vi "2D-square-lattice-generator.vi"(0 "index (row)":i32=150, 4 "Slope":dbl=41.0 format="%.2f", 5 "Period Y":dbl=333.0 format="%.2f", 6 "Spl Height":dbl=100.0 format="%.2f", 7 "Period X":dbl=329.0 format="%.2f", 8 "Width Y":dbl=200.0 format="%.2f", 9 "Width X":dbl=157.0 format="%.2f", 10 "Pixels Y":i32=1000, 11 "Pixels X":i32=1000) -> (1 "Sample Section":dbl[](graph)=[0.0, 0.0, 0.0, 0.0, 0.0, 0.0, 0.0, 0.0, 0.0, 0.0, 0.0, 0.0, 0.0, 0.0, 0.0, 0.0, 0.0, 0.0, 0.0, 0.0, 0.0, 0.0, 0.0, 0.0, 0.0, 0.0, 1.2195121951219523, 3.658536585365857, 6.0975609756097615, 8.536585365853655, 10.97560975609756, 13.414634146341465, 15.85365853658537, 18.292682926829272, 20.731707317073166, 23.17073170731707, 25.609756097560975, 28.04878048780488, 30.487804878048784, 32.92682926829268, 35.36585365853659, 37.80487804878049, 40.243902439024396, 42.6829268292683, 45.12195121951219, 47.5609756097561, 50.0, 52.4390243902439, 54.87804878048781, 57.31707317073172, 59.756097560975604, 62.19512195121951, 64.63414634146342, 67.07317073170731, 69.51219512195121, 71.95121951219512, 74.39024390243902, 76.82926829268293, 79.26829268292683, 81.70731707317074, 84.14634146341463, 86.58536585365853, 89.02439024390245, 91.46341463414635, 93.90243902439023, 96.34146341463415, 98.78048780487805, 100.0, 100.0, 100.0, 100.0, 100.0, 100.0, 100.0, 100.0, 100.0, 100.0, 100.0, 100.0, 100.0, 100.0, 100.0, 100.0, 100.0, 100.0, 100.0, 100.0, 100.0, 100.0, 100.0, 100.0, 100.0, 100.0, 100.0, 100.0, 100.0, 100.0, 100.0, 100.0, 100.0, 100.0, 100.0, 100.0, 100.0, 100.0, 100.0, 100.0, 100.0, 100.0, 100.0, 100.0, 100.0, 100.0, 100.0, 100.0, 100.0, 100.0, 100.0, 100.0, 100.0, 100.0, 100.0, 100.0, 100.0, 100.0, 100.0, 100.0, 100.0, 100.0, 100.0, 100.0, 100.0, 100.0, 100.0, 100.0, 100.0, 100.0, 100.0, 100.0, 100.0, 100.0, 100.0, 100.0, 100.0, 100.0, 100.0, 100.0, 100.0, 100.0, 100.0, 100.0, 100.0, 100.0, 100.0, 100.0, 100.0, 100.0, 100.0, 100.0, 100.0, 100.0, 100.0, 100.0, 100.0, 100.0, 100.0, 100.0, 100.0, 100.0, 100.0, 100.0, 100.0, 100.0, 100.0, 100.0, 100.0, 100.0, 100.0, 100.0, 100.0, 100.0, 100.0, 100.0, 100.0, 100.0, 100.0, 100.0, 100.0, 100.0, 100.0, 100.0, 100.0, 100.0, 100.0, 100.0, 100.0, 100.0, 100.0, 100.0, 100.0, 100.0, 100.0, 100.0, 100.0, 100.0, 100.0, 100.0, 100.0, 100.0, 100.0, 100.0, 100.0, 100.0, 100.0, 100.0, 100.0, 100.0, 100.0, 100.0, 100.0, 100.0, 100.0, 100.0, 100.0, 100.0, 100.0, 100.0, 100.0, 100.0, 100.0, 100.0, 100.0, 100.0, 100.0, 100.0, 100.0, 100.0, 100.0, 100.0, 100.0, 100.0, 100.0, 100.0, 100.0, 100.0, 100.0, 100.0, 100.0, 100.0, 100.0, 100.0, 100.0, 100.0, 100.0, 100.0, 100.0, 100.0, 100.0, 100.0, 100.0, 100.0, 100.0, 100.0, 100.0, 100.0, 100.0, 100.0, 98.78048780487805, 96.34146341463415, 93.90243902439023, 91.46341463414635, 89.02439024390245, 86.58536585365853, 84.14634146341463, 81.70731707317074, 79.26829268292683, 76.82926829268293, 74.39024390243902, 71.95121951219512, 69.51219512195121, 67.07317073170731, 64.63414634146342, 62.19512195121951, 59.756097560975604, 57.31707317073172, 54.87804878048781, 52.4390243902439, 50.0, 47.5609756097561, 45.12195121951219, 42.6829268292683, 40.243902439024396, 37.80487804878049, 35.36585365853659, 32.92682926829268, 30.487804878048784, 28.04878048780488, 25.609756097560975, 23.17073170731707, 20.731707317073166, 18.292682926829272, 15.85365853658537, 13.414634146341465, 10.97560975609756, 8.536585365853655, 6.0975609756097615, 3.658536585365857, 1.2195121951219523, 0.0, 0.0, 0.0, 0.0, 0.0, 0.0, 0.0, 0.0, 0.0, 0.0, 0.0, 0.0, 0.0, 0.0, 0.0, 0.0, 0.0, 0.0, 0.0, 0.0, 0.0, 0.0, 0.0, 0.0, 0.0, 0.0, 0.0, 0.0, 0.0, 0.0, 0.0, 0.0, 0.0, 0.0, 0.0, 0.0, 0.0, 0.0, 0.0, 0.0, 0.0, 0.0, 0.0, 0.0, 0.0, 0.0, 0.0, 0.0, 0.0, 0.0, 0.0, 1.2195121951219523, 3.658536585365857, 6.0975609756097615, 8.536585365853655, 10.97560975609756, 13.414634146341465, 15.85365853658537, 18.292682926829272, 20.731707317073166, 23.17073170731707, 25.609756097560975, 28.04878048780488, 30.487804878048784, 32.92682926829268, 35.36585365853659, 37.80487804878049, 40.243902439024396, 42.6829268292683, 45.12195121951219, 47.5609756097561, 50.0, 52.4390243902439, 54.87804878048781, 57.31707317073172, 59.756097560975604, 62.19512195121951, 64.63414634146342, 67.07317073170731, 69.51219512195121, 71.95121951219512, 74.39024390243902, 76.82926829268293, 79.26829268292683, 81.70731707317074, 84.14634146341463, 86.58536585365853, 89.02439024390245, 91.46341463414635, 93.90243902439023, 96.34146341463415, 98.78048780487805, 100.0, 100.0, 100.0, 100.0, 100.0, 100.0, 100.0, 100.0, 100.0, 100.0, 100.0, 100.0, 100.0, 100.0, 100.0, 100.0, 100.0, 100.0, 100.0, 100.0, 100.0, 100.0, 100.0, 100.0, 100.0, 100.0, 100.0, 100.0, 100.0, 100.0, 100.0, 100.0, 100.0, 100.0, 100.0, 100.0, 100.0, 100.0, 100.0, 100.0, 100.0, 100.0, 100.0, 100.0, 100.0, 100.0, 100.0, 100.0, 100.0, 100.0, 100.0, 100.0, 100.0, 100.0, 100.0, 100.0, 100.0, 100.0, 100.0, 100.0, 100.0, 100.0, 100.0, 100.0, 100.0, 100.0, 100.0, 100.0, 100.0, 100.0, 100.0, 100.0, 100.0, 100.0, 100.0, 100.0, 100.0, 100.0, 100.0, 100.0, 100.0, 100.0, 100.0, 100.0, 100.0, 100.0, 100.0, 100.0, 100.0, 100.0, 100.0, 100.0, 100.0, 100.0, 100.0, 100.0, 100.0, 100.0, 100.0, 100.0, 100.0, 100.0, 100.0, 100.0, 100.0, 100.0, 100.0, 100.0, 100.0, 100.0, 100.0, 100.0, 100.0, 100.0, 100.0, 100.0, 100.0, 100.0, 100.0, 100.0, 100.0, 100.0, 100.0, 100.0, 100.0, 100.0, 100.0, 100.0, 100.0, 100.0, 100.0, 100.0, 100.0, 100.0, 100.0, 100.0, 100.0, 100.0, 100.0, 100.0, 100.0, 100.0, 100.0, 100.0, 100.0, 100.0, 100.0, 100.0, 100.0, 100.0, 100.0, 100.0, 100.0, 100.0, 100.0, 100.0, 100.0, 100.0, 100.0, 100.0, 100.0, 100.0, 100.0, 100.0, 100.0, 100.0, 100.0, 100.0, 100.0, 100.0, 100.0, 100.0, 100.0, 100.0, 100.0, 100.0, 100.0, 100.0, 100.0, 100.0, 100.0, 100.0, 100.0, 100.0, 100.0, 100.0, 100.0, 100.0, 100.0, 100.0, 100.0, 100.0, 100.0, 100.0, 100.0, 100.0, 100.0, 100.0, 100.0, 100.0, 98.78048780487805, 96.34146341463415, 93.90243902439023, 91.46341463414635, 89.02439024390245, 86.58536585365853, 84.14634146341463, 81.70731707317074, 79.26829268292683, 76.82926829268293, 74.39024390243902, 71.95121951219512, 69.51219512195121, 67.07317073170731, 64.63414634146342, 62.19512195121951, 59.756097560975604, 57.31707317073172, 54.87804878048781, 52.4390243902439, 50.0, 47.5609756097561, 45.12195121951219, 42.6829268292683, 40.243902439024396, 37.80487804878049, 35.36585365853659, 32.92682926829268, 30.487804878048784, 28.04878048780488, 25.609756097560975, 23.17073170731707, 20.731707317073166, 18.292682926829272, 15.85365853658537, 13.414634146341465, 10.97560975609756, 8.536585365853655, 6.0975609756097615, 3.658536585365857, 1.2195121951219523, 0.0, 0.0, 0.0, 0.0, 0.0, 0.0, 0.0, 0.0, 0.0, 0.0, 0.0, 0.0, 0.0, 0.0, 0.0, 0.0, 0.0, 0.0, 0.0, 0.0, 0.0, 0.0, 0.0, 0.0, 0.0, 0.0, 0.0, 0.0, 0.0, 0.0, 0.0, 0.0, 0.0, 0.0, 0.0, 0.0, 0.0, 0.0, 0.0, 0.0, 0.0, 0.0, 0.0, 0.0, 0.0, 0.0, 0.0, 0.0, 0.0, 0.0, 0.0, 1.2195121951219523, 3.658536585365857, 6.0975609756097615, 8.536585365853655, 10.97560975609756, 13.414634146341465, 15.85365853658537, 18.292682926829272, 20.731707317073166, 23.17073170731707, 25.609756097560975, 28.04878048780488, 30.487804878048784, 32.92682926829268, 35.36585365853659, 37.80487804878049, 40.243902439024396, 42.6829268292683, 45.12195121951219, 47.5609756097561, 50.0, 52.4390243902439, 54.87804878048781, 57.31707317073172, 59.756097560975604, 62.19512195121951, 64.63414634146342, 67.07317073170731, 69.51219512195121, 71.95121951219512, 74.39024390243902, 76.82926829268293, 79.26829268292683, 81.70731707317074, 84.14634146341463, 86.58536585365853, 89.02439024390245, 91.46341463414635, 93.90243902439023, 96.34146341463415, 98.78048780487805, 100.0, 100.0, 100.0, 100.0, 100.0, 100.0, 100.0, 100.0, 100.0, 100.0, 100.0, 100.0, 100.0, 100.0, 100.0, 100.0, 100.0, 100.0, 100.0, 100.0, 100.0, 100.0, 100.0, 100.0, 100.0, 100.0, 100.0, 100.0, 100.0, 100.0, 100.0, 100.0, 100.0, 100.0, 100.0, 100.0, 100.0, 100.0, 100.0, 100.0, 100.0, 100.0, 100.0, 100.0, 100.0, 100.0, 100.0, 100.0, 100.0, 100.0, 100.0, 100.0, 100.0, 100.0, 100.0, 100.0, 100.0, 100.0, 100.0, 100.0, 100.0, 100.0, 100.0, 100.0, 100.0, 100.0, 100.0, 100.0, 100.0, 100.0, 100.0, 100.0, 100.0, 100.0, 100.0, 100.0, 100.0, 100.0, 100.0, 100.0, 100.0, 100.0, 100.0, 100.0, 100.0, 100.0, 100.0, 100.0, 100.0, 100.0, 100.0, 100.0, 100.0, 100.0, 100.0, 100.0, 100.0, 100.0, 100.0, 100.0, 100.0, 100.0, 100.0, 100.0, 100.0, 100.0, 100.0, 100.0, 100.0, 100.0, 100.0, 100.0, 100.0, 100.0, 100.0, 100.0, 100.0, 100.0, 100.0, 100.0, 100.0, 100.0, 100.0, 100.0, 100.0, 100.0, 100.0, 100.0, 100.0, 100.0, 100.0, 100.0, 100.0, 100.0, 100.0, 100.0, 100.0, 100.0, 100.0, 100.0, 100.0, 100.0, 100.0, 100.0, 100.0, 100.0, 100.0, 100.0, 100.0, 100.0, 100.0, 100.0, 100.0, 100.0, 100.0, 100.0, 100.0, 100.0, 100.0, 100.0, 100.0, 100.0, 100.0, 100.0, 100.0, 100.0, 100.0, 100.0, 100.0, 100.0, 100.0, 100.0, 100.0, 100.0, 100.0, 100.0, 100.0, 100.0, 100.0, 100.0, 100.0, 100.0, 100.0, 100.0, 100.0, 100.0, 100.0, 100.0, 100.0, 100.0, 100.0, 100.0, 100.0, 100.0, 100.0, 100.0, 100.0, 100.0, 100.0, 100.0, 98.78048780487805, 96.34146341463415, 93.90243902439023, 91.46341463414635, 89.02439024390245, 86.58536585365853, 84.14634146341463, 81.70731707317074, 79.26829268292683, 76.82926829268293, 74.39024390243902, 71.95121951219512, 69.51219512195121, 67.07317073170731, 64.63414634146342, 62.19512195121951, 59.756097560975604, 57.31707317073172, 54.87804878048781, 52.4390243902439, 50.0, 47.5609756097561, 45.12195121951219, 42.6829268292683, 40.243902439024396, 37.80487804878049, 35.36585365853659, 32.92682926829268, 30.487804878048784, 28.04878048780488, 25.609756097560975, 23.17073170731707, 20.731707317073166, 18.292682926829272, 15.85365853658537, 13.414634146341465, 10.97560975609756, 8.536585365853655, 6.0975609756097615, 3.658536585365857, 1.2195121951219523, 0.0, 0.0, 0.0, 0.0, 0.0, 0.0, 0.0, 0.0, 0.0, 0.0, 0.0, 0.0, 0.0, 0.0, 0.0, 0.0, 0.0, 0.0, 0.0, 0.0, 0.0, 0.0, 0.0, 0.0, 0.0, 0.0], 2 "2D Sample":dbl[][](graph))   [LabVIEW 2017]
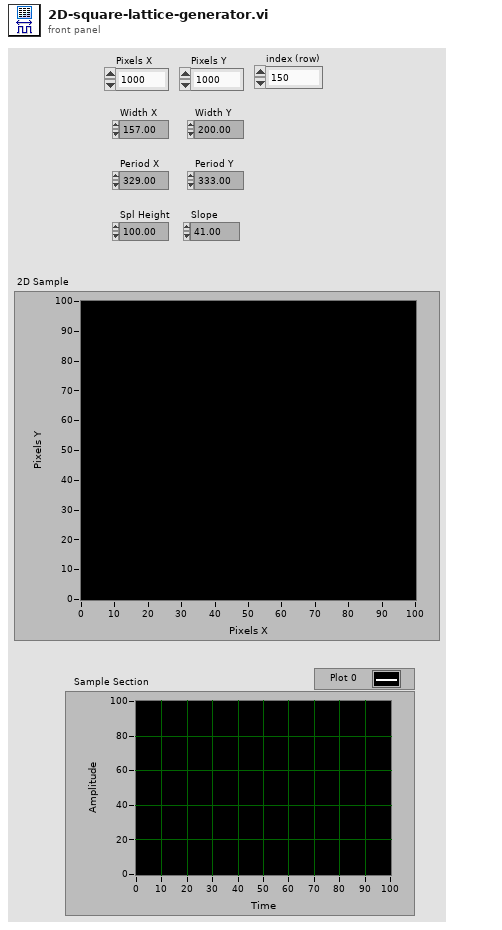
[diagram p1: front panel]
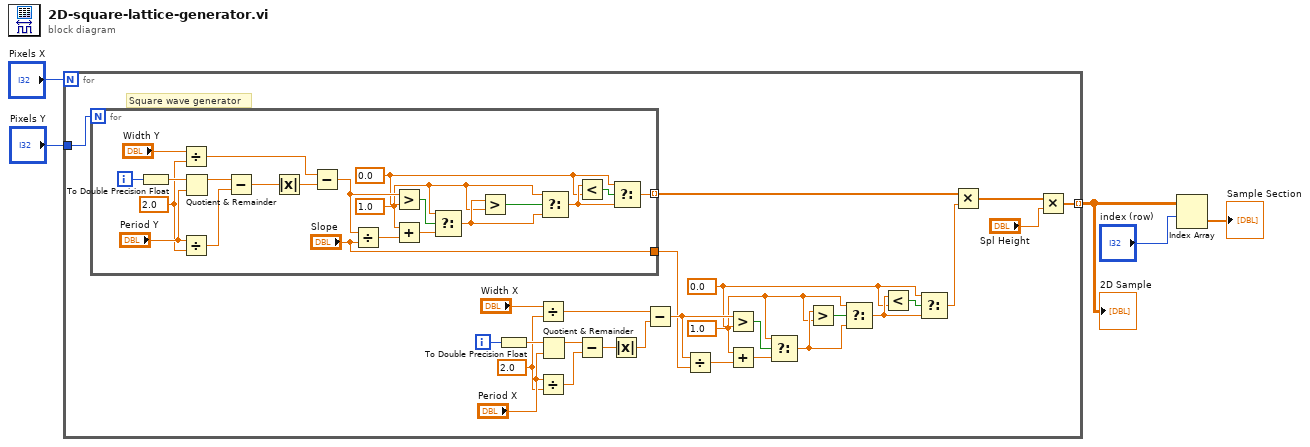
[diagram p0: block diagram]
diagram:
  n1 = for {
    N: "Pixels X" -> [_]
    tunnel: "Pixels Y" -> [w32]
    tunnel: [w6] -> w3 mode=indexing
    i -> [w12]
    w13 = 0.0 ("t")
    w14 = 1.0 ("t")
    w15 = 2.0 ("y")
    # "Square wave generator"
    n2 = for {
      N: w32 -> [_]
      tunnel: ["Slope"] -> w11
      tunnel: [w33] -> w9 mode=indexing
      i -> [w54]
      w35 = 0.0 ("t")
      w36 = 1.0 ("t")
      w37 = 2.0 ("y")
      n3 = To Double Precision Float(number=w54) -> (double precision float=w38:dbl)
      n4 = Divide(x="Width Y", y=w37) -> (x/y=w44:dbl)
      n5 = Divide(x="Period Y", y=w37) -> (x/y=w48:dbl)
      n6 = Quotient & Remainder(x=w38, y="Period Y") -> (x-y*floor(x/y)=w49:dbl)  [unwired: 1 out]
      n7 = Subtract(x=w49, y=w48) -> (x-y=w47:dbl)
      n8 = Absolute Value(x=w47) -> (abs(x)=w45:dbl)
      n9 = Subtract(x=w44, y=w45) -> (x-y=w42:dbl)
      n10 = Divide(x=w42, y="Slope") -> (x/y=w41:dbl)
      n11 = Greater?(x=w42, y=w35) -> (0:w43:bool)
      n12 = Add(x=w36, y=w41) -> (x+y=w40:dbl)
      n13 = Select(t=w36, s=w43, f=w40) -> (s? t:f=w39:dbl)
      n14 = Greater?(x=w39, y=w36) -> (0:w52:bool)
      n15 = Select(t=w36, s=w52, f=w39) -> (s? t:f=w50:dbl)
      n16 = Less?(x=w50, y=w35) -> (x < y?=w51:bool)
      n17 = Select(t=w35, s=w51, f=w50) -> (s? t:f=w33:dbl)
    }
    n18 = To Double Precision Float(number=w12) -> (double precision float=w16:dbl)
    n19 = Divide(x="Width X", y=w15) -> (x/y=w22:dbl)
    n20 = Divide(x="Period X", y=w15) -> (x/y=w26:dbl)
    n21 = Quotient & Remainder(x=w16, y="Period X") -> (x-y*floor(x/y)=w27:dbl)  [unwired: 1 out]
    n22 = Subtract(x=w27, y=w26) -> (x-y=w25:dbl)
    n23 = Absolute Value(x=w25) -> (abs(x)=w23:dbl)
    n24 = Subtract(x=w22, y=w23) -> (x-y=w20:dbl)
    n25 = Divide(x=w20, y=w11) -> (x/y=w19:dbl)
    n26 = Greater?(x=w20, y=w13) -> (0:w21:bool)
    n27 = Add(x=w14, y=w19) -> (x+y=w18:dbl)
    n28 = Select(t=w14, s=w21, f=w18) -> (s? t:f=w17:dbl)
    n29 = Greater?(x=w17, y=w14) -> (0:w30:bool)
    n30 = Select(t=w14, s=w30, f=w17) -> (s? t:f=w28:dbl)
    n31 = Less?(x=w28, y=w13) -> (x < y?=w29:bool)
    n32 = Select(t=w13, s=w29, f=w28) -> (s? t:f=w10:dbl)
    n33 = Multiply(x=w9, y=w10) -> (x*y=w8:dbl[])
    n34 = Multiply(x=w8, y="Spl Height") -> (x*y=w6:dbl[])
  }
  "2D Sample" <- w3
  n35 = Index Array(array=w3, index (row)="index (row)") -> (element=→"Sample Section":dbl[])  [unwired: 1 in]
